vi "PPMS Build Self Extracting Installer.vi"(8 "Path to project":path=path "C:/Users/patrick/Documents/GitHub/levylabpitt/PPMS-Monitor-and-Control/PPMS_inst.lvproj", 9 "Package Version":string="2.0.0.6") -> (0 "Error Out":errorcluster)   [LabVIEW 2019]
uses:
  <userlib>/LevyLab/Build Support/PostBuildSupport/PostBuildSupport.lvclass
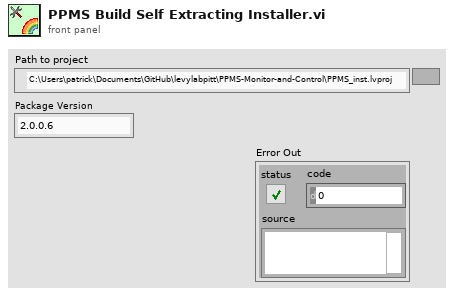
[diagram p1: front panel]
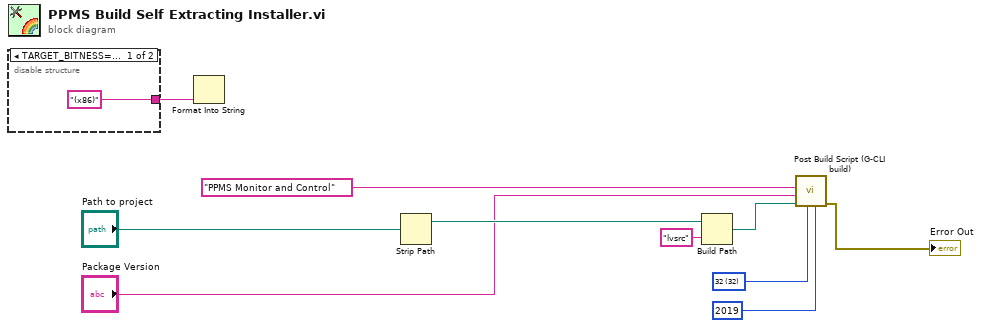
[diagram p0: block diagram]
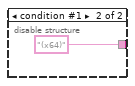
[diagram p2: hidden frame]
diagram:
  w2 = u32 32 items=["32"=32, "64"=64] ("Architecture")
  n1 = disable-structure shown="TARGET_BITNESS==32, Default" {
    disable-tunnel: ["(x86)" ("Name of build specification") "(x64)" ("Name of build specification")] -> w10
    frame condition #0 (active) {
    }
    frame condition #1 {
    }
  }
  n2 = Format Into String(w10) -> ()  [unwired: 3 in, 2 out]
  n3 = Strip Path(path="Path to project") -> (stripped path=w9:path)  [unwired: 1 out]
  n4 = Build Path(base path=w9, name or relative path="lvsrc") -> (appended path=w3:path)
  n5 = call <userlib>:"Post Build Script (G-CLI build).vi"("LV Version"=u32 2019, "Architecture"=w2, "Package Source Folder"=w3, "Package Version"="Package Version", "Product Name"="PPMS Monitor and Control") -> ("error out"=→"Error Out":errorcluster)  [unwired: 6 in]
